vi "SnakeGameControlAdapter.vi"(8 "error in (no error)":errorcluster, 11 "Controller in":refnum<class "Controller.lvclass">) -> (0 "error out":errorcluster, 3 "Controller out":refnum<class "Controller.lvclass">)   [LabVIEW 2014, in "Controller.lvclass"]
uses:
  Controller.lvclass
  TypeDefs/SnakeMovements.ctl
panel:
  out "Movement":T1
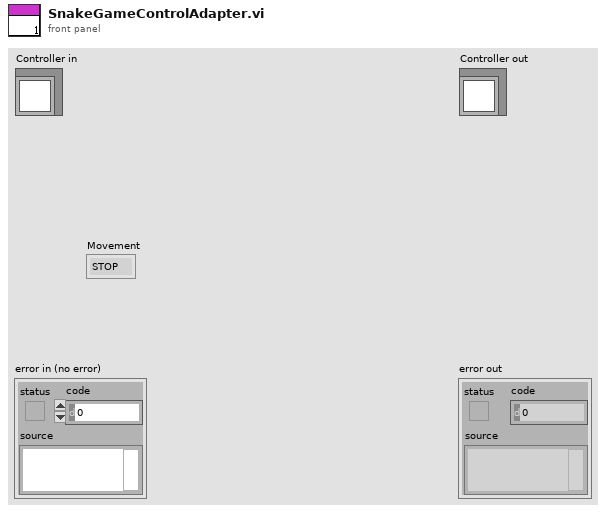
[diagram p1: front panel]
types:
  T1 = typedef "SnakeMovements.ctl" = enum16{"STOP", "UP", "DOWN", "RIGHT", "LEFT"}
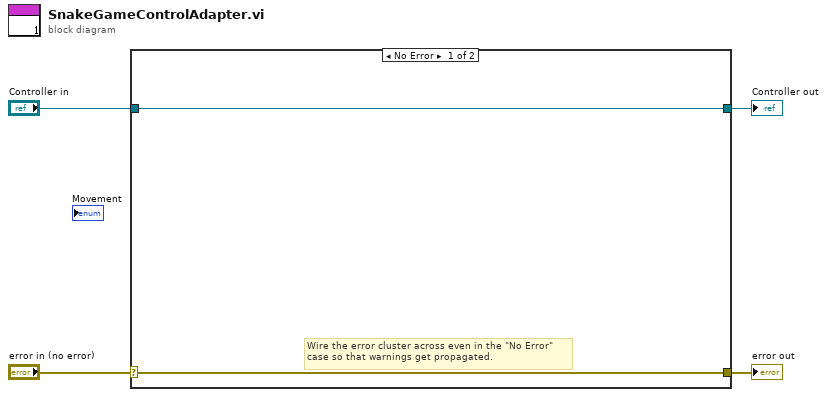
[diagram p0: block diagram]
diagram:
  n1 = case shown="No Error" "error in (no error)" {
    selector: "error in (no error)" -> [w5 w8]
    tunnel: [w5 w8] -> w3
    tunnel: [w6 w7] -> w1
    tunnel: "Controller in" -> [w6 w7]
    frame No Error {
      # "Wire the error cluster across even in the \"No Error\"\ncase so that warnings get propagated."
    }
    frame Error {
    }
  }
  "error out" <- w3
  "Controller out" <- w1
